vi "Monitor Demo.vi"() -> ()   [LabVIEW 2020]
uses:
  Flex/Flex.lvlib
panel:
  out "Stalled":bool
  out "Actual":u32
  out "Lossless 50mS":dbl(graph)
  out "Lossless 20mS":dbl(graph)
  out "Lossless 5mS":dbl(graph)
  in  "Stop":bool
  in  "Period mS":u32=20
  out "Buffers":dbl[](array[slide]) scale=0.0..1.0
  in  "Slide":dbl(slide) scale=0.0..10.0
  out "Count":i32[](array[numeric])
  # "Producer"
  # "The order of consumers can be random in these indicators"
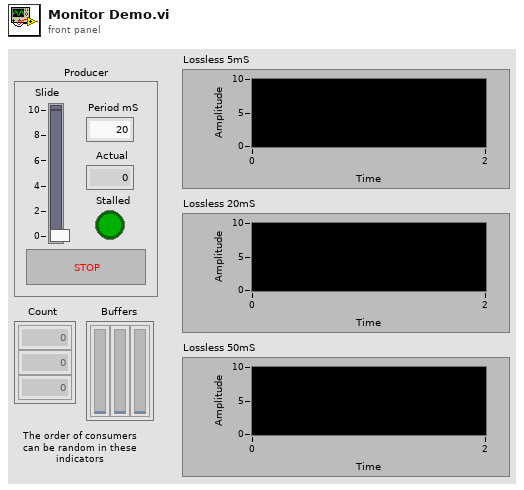
[diagram p1: front panel]
types:
  T1 = typedef "Flex.lvlib/))Channel.ctl" = refnum<queue>
  T2 = typedef "Flex.lvlib/Element.ctl" = dbl
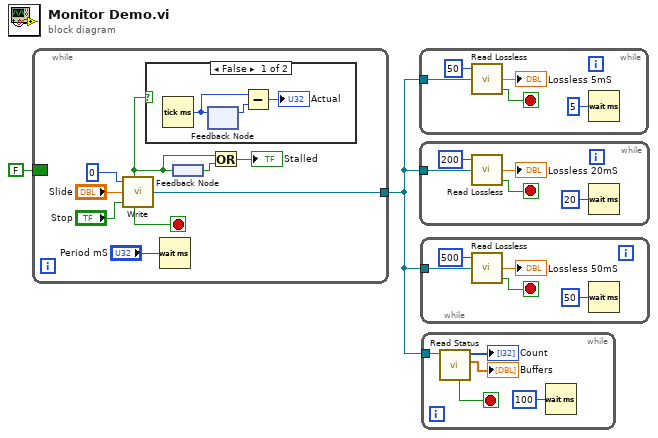
[diagram p0: block diagram]
diagram:
  n1 = while {
    tunnel: [w8] -> w2
    border: FALSE ("Timed Out?") -> [_]
    stop <- w7 stop-if-true
    n2 = call "Write.vi"("Timeout mS (-1)"=0, "element"="Slide", "Close? (F)"="Stop") -> ("Timed Out?"=w3:bool, "Closed?"=w7:bool, "channel"=w8:T1)  [unwired: 2 in]
    n3 = case shown="False" w3 {
      frame False {
        n4 = Tick Count (ms)() -> (millisecond timer value=w13:u32)
        n5 = feedback #1() -> (w12:u32)  [unwired: 1 in]
        n6 = feedback-in #1(w13) -> ()
        n7 = Subtract(x=w13, y=w12) -> (x-y=→"Actual":u32)
      }
      frame True {
      }
    }
    n8 = Wait (ms)(milliseconds to wait="Period mS") -> ()  [unwired: 1 out]
    n9 = feedback #2() -> (w5:bool)
    n10 = feedback-in #2(w3) -> ()
    n11 = Or(x=w3, y=w5) -> (x .or. y?=→"Stalled":bool)
  }
  n12 = while {
    tunnel: w2 -> [w19]
    stop <- w17 stop-if-true
    n13 = call "Read Lossless.vi"("Depth (Unlimited)"=50, "FlexChannel"=w19) -> ("Element"=→"Lossless 5mS":T2, "Closed?"=w17:bool)  [unwired: 5 in, 1 out]
    n14 = Wait (ms)(milliseconds to wait=u32 5) -> ()  [unwired: 1 out]
  }
  n15 = while {
    tunnel: w2 -> [w24]
    stop <- w22 stop-if-true
    n16 = call "Read Lossless.vi"("Depth (Unlimited)"=200, "FlexChannel"=w24) -> ("Element"=→"Lossless 20mS":T2, "Closed?"=w22:bool)  [unwired: 5 in, 1 out]
    n17 = Wait (ms)(milliseconds to wait=u32 20) -> ()  [unwired: 1 out]
  }
  n18 = while {
    tunnel: w2 -> [w29]
    stop <- w27 stop-if-true
    n19 = call "Read Lossless.vi"("Depth (Unlimited)"=500, "FlexChannel"=w29) -> ("Element"=→"Lossless 50mS":T2, "Closed?"=w27:bool)  [unwired: 5 in, 1 out]
    n20 = Wait (ms)(milliseconds to wait=u32 50) -> ()  [unwired: 1 out]
  }
  n21 = while {
    tunnel: w2 -> [w33]
    stop <- w32 stop-if-true
    n22 = call "Read Status.vi"("channel"=w33) -> ("Usage Ratio"=→"Buffers":dbl[], "Queued Count"=→"Count":i32[], "Closed?"=w32:bool)  [unwired: 4 in, 4 out]
    n23 = Wait (ms)(milliseconds to wait=u32 100) -> ()  [unwired: 1 out]
  }
